vi "获取索引.vi"(8 "error in (no error)":errorcluster caption="错误输入（无错误）", 11 "程序 输入":refnum<class "程序.lvclass">) -> (0 "error out":errorcluster caption="错误输出", 3 "程序 输出":refnum<class "程序.lvclass">)   [LabVIEW 2020, in "程序.lvclass"]
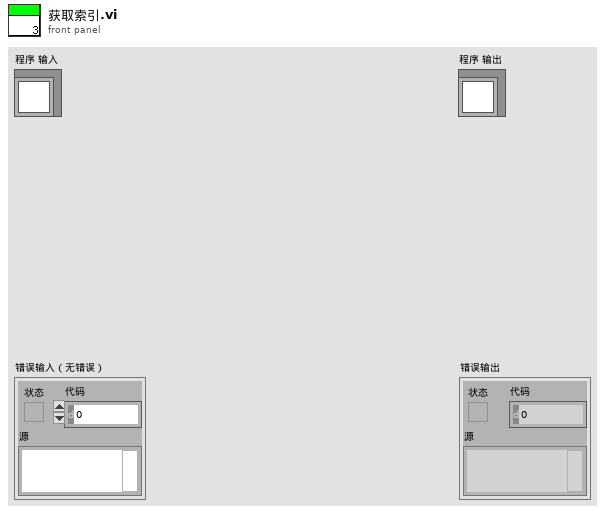
[diagram p1: front panel]
types:
  T1 = typedef "LVPoint32TypeDef.ctl" = cluster{"Horizontal":i32, "Vertical":i32}
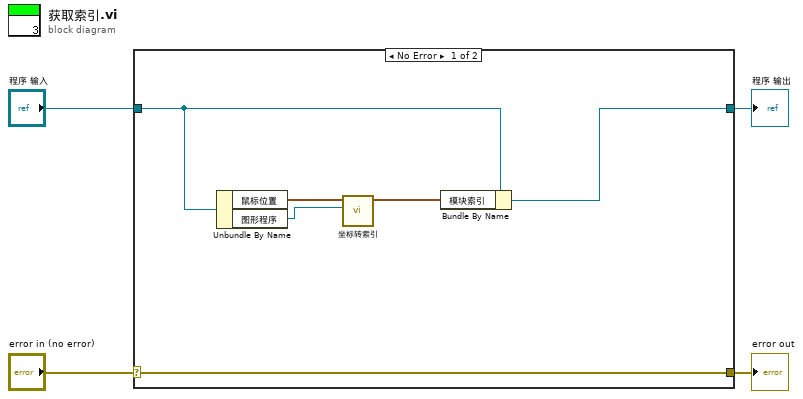
[diagram p0: block diagram]
diagram:
  n1 = case shown="No Error" "error in (no error)" {
    selector: "error in (no error)" -> [w10 w12]
    tunnel: [w10 w12] -> w3
    tunnel: [w5 w11] -> w1
    tunnel: "程序 输入" -> [w6 w11]
    frame No Error {
      n2 = Unbundle By Name(w6) -> ("鼠标位置"=w9:T1, "图形程序"=w8:refnum<vi>)
      n3 = call "坐标转索引.vi"("图形程序"=w8, "坐标"=w9) -> ("索引"=w7:cluster{"列":i32, "行":i32})  [unwired: 9 in]
      n4 = Bundle By Name(cluster=w6, "模块索引"=w7) -> (w5:refnum<class "程序.lvclass">)
    }
    frame Error {
    }
  }
  "error out" <- w3
  "程序 输出" <- w1
